vi "SVFA FFT Spectrum Subset (Mag-Phase) (N Ch).vi"(0 "scaled signals [EU]":waveform(dbl)[](array[waveform]), 2 "window":T1=1 items=["None"=0, "Hanning"=1, "Hamming"=2, "Blackman-Harris"=3, "Exact Blackman"=4, "Blackman"=5, "Flat Top"=6, "4 Term B-Harris "=7, "7 Term B-Harris"=8, "Low Sidelobe"=9, "Force"=64, "Exponential"=65, "Blackman Nuttall"=11, "Triangle"=30, "Bartlett-Hanning"=31, "Bohman"=32, "Parzen"=33, "Welch"=34, "Kaiser"=60, "Dolph-Chebyshev"=61, "Gaussian"=62], 3 "frequency range":T3={"start frequency"=1000.0, "stop frequency"=5000.0} {"stop frequency" min=0.0 format="%.2f"; "start frequency" min=0.0 format="%.2f"}, 4 "view":T2={"dB On (T)"=TRUE, "unwrap phase (F)"=FALSE, "convert to degree (T)"=TRUE}, 5 "error in (no error)":errorcluster, 7 "averaging parameters":T10={"averaging mode"=enum."No averaging", "weighting mode"=enum."Exponential", "number of averages"=10, "linear mode"=enum."One shot"} {"number of averages" min=1 step=1}, 9 "restart averaging (F)":bool) -> (11 "averaging done":bool, 13 "averages completed":dbl, 14 "magnitudes [dB EU]":cluster{"f0":dbl, "df":dbl, "magnitude":dbl[]}[](array[cluster]) {"magnitude" format="%.2p"; "df" format="%.2p"; "f0" format="%.2p"}, 15 "magnitude unit labels":string[](array[string]), 16 "phases [degrees]":cluster{"f0":dbl, "df":dbl, "phase":dbl[]}[](array[cluster]) {"phase" format="%.2f"; "df" format="%.2f"; "f0" format="%.2f"}, 17 "phase unit labels":string[](array[string]), 18 "spectrum info":T4[](array[typedef]) {"x-axis units" items=["Time (s)"=0, "Frequency-CB (Hz)"=1, "Frequency-CPB (Hz)"=1248, "Frequency-Arbitrary (Hz)"=2357, "Quefrency (s)"=2, "Revolutions (rev)"=3, "Order"=4, "Speed (RPM)"=11, "Speed (rad/s)"=21, "Index"=65535]; "weighting filter" items=["Linear", "A-weighting", "B-weighting", "C-weighting", "ITU-R 468-4", "Dolby", "CCITT", "C-message", "Wb", "Wc", "Wd", "We", "Wf", "Wh", "Wj", "Wk", "Wm", "AES17 20 kHz lowpass", "AES17 40 kHz lowpass", "AES17 20 kHz highpass", "AES17 40 kHz highpass"]; "dB reference [EU]" format="%.2f"; "engineering units" items=["custom..."=0, "V"=1, "A"=21, "C"=30, "pC"=31, "s"=32, "-"=29, "Pa"=2, "N"=20, "g"=3, "m/s^2"=4, "m/s"=5, "m"=6, "mm/s"=12, "mm"=13, "micron/s"=14, "micron"=15, "in/s^2"=7, "in/s"=8, "in"=9, "mil/s"=10, "mil"=11, "rad/s^2"=16, "rad/s"=17, "rad"=18, "deg/s^2"=26, "deg/s"=27, "deg"=28, "RPM"=22, "cycle/s^2"=23, "Hz"=24, "cycle"=25, "strain"=19]; "spectral info"."window" items=["None "=0, "Hanning"=1, "Hamming"=2, "Blackman-Harris"=3, "Exact Blackman"=4, "Blackman"=5, "Flat Top"=6, "4 Term B-Harris "=7, "7 Term B-Harris"=8, "Low Sidelobe"=9, "Force - Exponential"=10, "Gaussian"=62]}, 19 "error out":errorcluster)   [LabVIEW 2017]
doc: "Computes a subset of the FFT spectrum of <B>scaled signal [EU]</B>. The subset is defined by <B>frequency range</B>. FFT results are returned as magnitude and phase. Each block of data corresponds to a single FFT block and has to be passed individually to this VI. Wire data to the <B>scaled signal [EU]</B> input to determine the polymorphic instance to use or manually select the instance."
uses:
  <vilib>/addons/_NISVFA/_Shared subVIs/Controls/svc_Spectrum Info.ctl
  <vilib>/addons/_NISVFA/_Shared subVIs/Controls/svc_X-Axis Units.ctl
  <vilib>/addons/_NISVFA/_Shared subVIs/Controls/svc_Spectrum Type.ctl
  <vilib>/addons/_NISVFA/_Shared subVIs/Controls/svc_Engineering Units Text Ring.ctl
  <vilib>/addons/_NISVFA/_Shared subVIs/Controls/svc_Weighting Filter Text Ring.ctl
  <vilib>/addons/_NISVFA/_Shared subVIs/Controls/svc_Complimentary Spectrum Units.ctl
  <vilib>/addons/_NISVFA/_Shared subVIs/Controls/svc_Window.ctl
  <vilib>/addons/_NISVFA/_Shared subVIs/Windowing/svfa_Scaled Time Domain Window (1 Ch).vi
  <vilib>/addons/_NISVFA/_Shared subVIs/Spectrum Info/svfa_Build Spectrum Info.vi
  <vilib>/addons/_NISVFA/_Shared subVIs/Spectrum Averaging/svfa_Reset Averaging State Info.vi
  <vilib>/addons/_NISVFA/_Shared subVIs/Spectrum Averaging/svfa_Average Array with Avg Checks (complex) No State.vi
  <vilib>/addons/_NISVFA/_Shared subVIs/Common/svc_Complex to Mag2 Array.vi
  <vilib>/addons/_NISVFA/_Shared subVIs/Spectrum Averaging/svfa_Average Array with Avg Checks (real) No State.vi
  <vilib>/addons/_NISVFA/_Shared subVIs/Windowing/svfa_Scaled Time Domain Window (Array).vi
  <vilib>/addons/_NISVFA/_Shared subVIs/Common/svc_Get SV Channel Info.vi
  <vilib>/addons/_NISVFA/_Shared subVIs/Common/svc_Spectrum Units.vi
  <vilib>/addons/_NISVFA/_Shared subVIs/Spectrum Averaging/svfa_Average Array (complex) No State.vi
  <vilib>/addons/_NISVFA/_Shared subVIs/Spectrum Averaging/svfa_Average Array (real) No State.vi
  <vilib>/Analysis/4window.llb/Force Window.vi
  <vilib>/Analysis/4window.llb/Force Window (DBL).vi
  <vilib>/Analysis/4window.llb/Exponential Window.vi
  <vilib>/Analysis/4window.llb/Exponential Window (DBL).vi
  <vilib>/addons/_NISVFA/_Shared subVIs/Spectrum Averaging/svfa_No Average Array (complex).vi
  <vilib>/addons/_NISVFA/_Shared subVIs/Spectrum Averaging/svfa_Average Array (complex).vi
  <vilib>/addons/_NISVFA/_Shared subVIs/Spectrum Averaging/svfa_No Average Array (real).vi
  <vilib>/addons/_NISVFA/_Shared subVIs/Spectrum Averaging/svfa_Average Array (real).vi
  <vilib>/addons/_NISVFA/_Shared subVIs/Spectrum Averaging/svfa_Peak Hold Array.vi
  <vilib>/addons/_NISVFA/_Shared subVIs/Common/svc_Get Weighting Enum and Labels.vi
  <vilib>/addons/_NISVFA/_Shared subVIs/Common/svc_Unit Label Lexical Class.vi
  <vilib>/addons/_NISVFA/_Shared subVIs/Common/svc_Engineering Units to Unit Label.vi
  <vilib>/addons/_NISVFA/_Shared subVIs/Common/svc_Format Value (DBL).vi
  <vilib>/addons/_NISVFA/_Shared subVIs/Common/svc_Channel Info to Spectrum Info.vi
  <vilib>/addons/_NISVFA/_Shared subVIs/Common/svc_Unit Label to Engineering Units.vi
  <vilib>/Utility/error.llb/Error Cluster From Error Code.vi
  <vilib>/Analysis/0measdsp.llb/Scaled Time Domain Window.vi
  <vilib>/Analysis/0measdsp.llb/Scaled Time Domain Window (DBL).vi
  <vilib>/addons/_NISVFA/_Spectrum Processing/subVIs/svfa_Spectrum Info Window to windowTd Type Def.vi
  <vilib>/addons/_NISVFA/_Shared subVIs/Common/svc_Window Parameters.vi
  <vilib>/addons/_NISVFA/_Shared subVIs/Common/svc_Get Window Info.vi
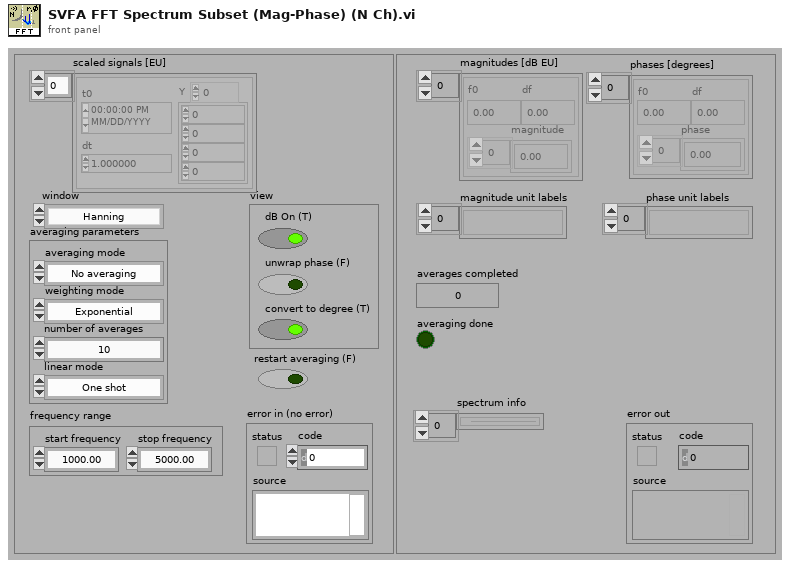
[diagram p1: front panel]
types:
  T1 = typedef "svc_Window.ctl" = u32
  T2 = cluster{"dB On (T)":bool, "unwrap phase (F)":bool, "convert to degree (T)":bool}
  T3 = cluster{"start frequency":dbl, "stop frequency":dbl}
  T4 = typedef "svc_Spectrum Info.ctl" = cluster{"channel name":string, "description":string, "x-axis units":T5, "spectral info":cluster{"spectrum type":T6, "linear/dB":enum16{"linear", "dB"}, "window":u16, "window size":i32, "FFT size":i32}, "engineering units":T7, "custom label":string, "dB reference [EU]":dbl, "peak units":enum16{"rms", "peak", "peak-peak"}, "weighting filter":T8, "spectral density?":bool, "unit label":string, "spectrum skewed?":bool, "complimentary spectrum units":T9}
  T5 = typedef "svc_X-Axis Units.ctl" = u16
  T6 = typedef "svc_Spectrum Type.ctl" = enum16{"FFT Spectrum [complex]", "Amplitude [Magnitude]", "Power [Magnitude^2]", "Cross Spectrum [complex]", "Frequency Response [Complex]"}
  T7 = typedef "svc_Engineering Units Text Ring.ctl" = u16
  T8 = typedef "svc_Weighting Filter Text Ring.ctl" = u16
  T9 = typedef "svc_Complimentary Spectrum Units.ctl" = enum16{"none", "radians", "degrees", "cycles", "imaginary"}
  T10 = cluster{"averaging mode":enum16{"No averaging", "Vector averaging", "RMS averaging", "Peak hold"}, "weighting mode":enum16{"Linear", "Exponential"}, "number of averages":u32, "linear mode":enum16{"One shot", "Auto restart"}}
  T11 = enum16{"Restart processing", "Continue processing", "Skip processing"}
  T12 = cluster{"complex FFT":cdb[], "real FFT":dbl[], "f0":dbl, "df":dbl, "averages completed":dbl, "averaging parameters":cluster{"averaging mode":enum16{"No averaging", "Vector averaging", "RMS averaging", "Peak hold"}, "weighting mode":enum16{"Linear", "Exponential"}, "number of averages":u32, "linear mode":enum16{"One shot", "Auto restart"}}}
  T13 = cluster{"complex FFT":cdb[], "real FFT":dbl[], "f0":dbl, "df":dbl, "averages completed":dbl, "averaging parameters":cluster{"averaging mode":enum16{"No averaging", "Vector averaging", "RMS averaging", "Peak hold"}, "weighting mode":enum16{"Linear", "Exponential"}, "number of averages":u32, "linear mode":enum16{"One shot", "Auto restart"}}}[]
  T14 = enum16{"No averaging", "Vector averaging", "RMS averaging", "Peak hold"}
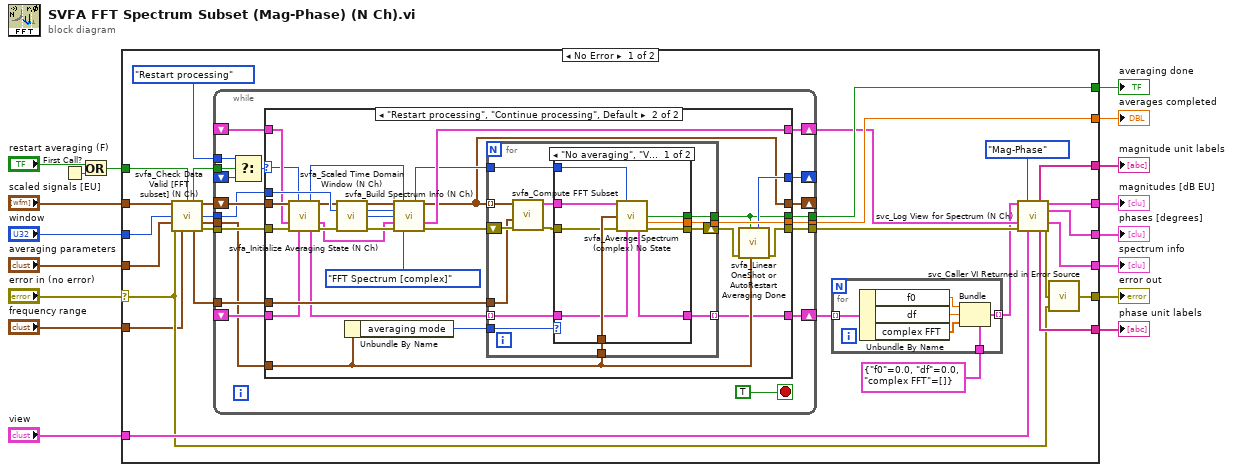
[diagram p0: block diagram]
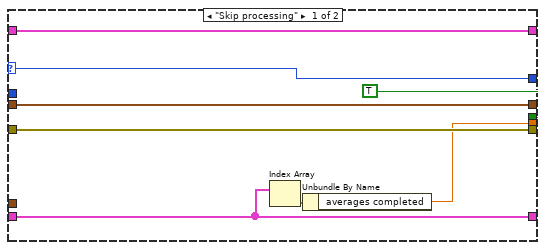
[diagram p2: hidden frame]
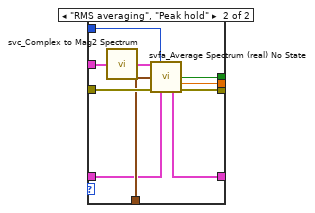
[diagram p3: hidden frame]
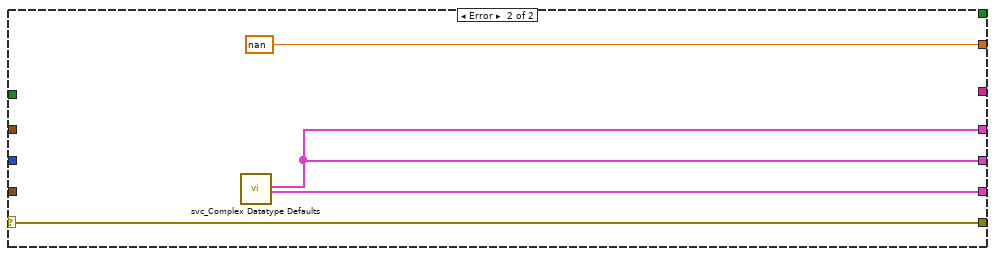
[diagram p4: hidden frame]
diagram:
  n1 = First Call?() -> (First Call?: T/F=w4:bool)
  n2 = Or(x="restart averaging (F)", y=w4) -> (x .or. y?=w2:bool)
  n3 = case shown="No Error" "error in (no error)" {
    selector: "error in (no error)" -> [w35 w144]
    tunnel: w2 -> [w41 _]
    tunnel: [w22 nan ("Averaged So-far")] -> w17
    tunnel: [w36 w144] -> w16
    tunnel: "averaging parameters" -> [w44 _]
    tunnel: "frequency range" -> [w32 _]
    tunnel: "scaled signals [EU]" -> [w46 _]
    tunnel: [w37 w141] -> w5
    tunnel: [w42 _] -> w11
    tunnel: [w45 _] -> w10
    tunnel: [w39 w142] -> w9
    tunnel: [w40 w142] -> w8
    tunnel: [w23 _] -> w7
    tunnel: "view" -> [w43 _]
    tunnel: "window" -> [w34 _]
    frame No Error {
      n4 = call <vilib>:"svfa_Check Data Valid [FFT subset] (N Ch).vi"("scaled signals"=w46, "restart averaging (F)"=w41, "window"=w34, "averaging parameters"=w44, "error in (no error)"=w35, "frequency range in"=w32) -> ("restart averaging"=w25:bool, "dup scaled signals"=w30:waveform(dbl)[], "window"=w29:u16, "dup averaging parameters"=w28:T10, "frequency range out"=w24:T3, "error out"=w27:errorcluster)  [unwired: 4 in]
      n5 = while {
        shift-left: _ -> [w63]
        shift-right: [w64] -> w31
        tunnel: w24 -> [w66]
        tunnel: [w68] -> w22
        tunnel: [w70] -> w23
        tunnel: w27 -> [w71]
        tunnel: [w69] -> w20
        tunnel: w29 -> [w59]
        tunnel: w28 -> [w58]
        shift-right: [w61] -> w21
        shift-left: _ -> [w60]
        shift-right: [w65] -> _
        shift-left: _ -> [w57]
        tunnel: T11."Restart processing" ("t") -> [w56]
        tunnel: w25 -> [w54]
        shift-right: [w53] -> _
        shift-left: w30 -> [w67]
        stop <- TRUE stop-if-true
        n6 = Select(t=w56, s=w54, f=w57) -> (s? t:f=w55:T11)
        n7 = case shown="\"Restart processing\", \"Continue processing\", Default" w55 {
          selector: w55 -> [w77 w82]
          tunnel: w58 -> [_ w106]
          tunnel: [w76 w100] -> w64
          tunnel: w67 -> [w72 w90]
          tunnel: w66 -> [_ w92]
          tunnel: [w77 w105] -> w65
          tunnel: w63 -> [w76 w87]
          tunnel: w59 -> [_ w107]
          tunnel: [w73 w93] -> w61
          tunnel: w60 -> [w73 w89]
          tunnel: [TRUE ("averaging done?") w102] -> w70
          tunnel: [w74 w108] -> w68
          tunnel: [w78 w104] -> w69
          tunnel: w71 -> [w78 w85]
          tunnel: [w72 w80] -> w53
          frame "Skip processing" {
            n8 = Index Array(array=w76) -> (element=w75:T12)  [unwired: 1 in]
            n9 = Unbundle By Name(w75) -> ("averages completed"=w74:dbl)
          }
          frame "Restart processing", "Continue processing", Default {
            n10 = call <vilib>:"svfa_Initialize Averaging State (N Ch).vi"("Windowed Waveform(s)"=w90, "processing control in"=w82, "spectra info in"=w89, "error in (no error)"=w85, "state info"=w87) -> ("processing control out"=w81:T11, "Windowed Waveform(s)"=w88:waveform(dbl)[], "spectra info out"=w83:T4[], "state info"=w86:T13, "error out"=w84:errorcluster)  [unwired: 6 in]
            n11 = call <vilib>:"svfa_Scaled Time Domain Window (N Ch).vi"("Scaled signal(s)"=w88, "window"=w107, "error in (no error)"=w84) -> ("Windowed Waveform(s)"=w97:waveform(dbl)[], "window"=w95:T1, "window length"=w96:i32, "error out"=w98:errorcluster)  [unwired: 8 in, 1 out]
            n12 = Unbundle By Name(w106) -> ("averaging mode"=w101:T14)
            n13 = call <vilib>:"svfa_Build Spectrum Info (N Ch).vi"("scaled signal(s)"=w97, "processing control in"=w81, "window"=w95, "window size"=w96, "spectra info in"=w83, "error in (no error)"=w98, "spectrum type"=svc_Spectrum_Type."FFT Spectrum [complex]" ("spectrum type 2")) -> ("dup processing control"=w91:T11, "dup scaled signals"=w80:waveform(dbl)[], "spectra info out"=w93:T4[], "error out"=w99:errorcluster)  [unwired: 5 in]
            n14 = for {
              tunnel: [w121] -> w108
              tunnel: w106 -> [w120]
              tunnel: [w118] -> w102
              tunnel: w101 -> [w117]
              tunnel: [w116] -> w100 mode=indexing
              tunnel: w92 -> [w114]
              tunnel: w91 -> [w111]
              tunnel: w80 -> [w110] mode=indexing
              tunnel: w86 -> [w109] mode=indexing
              shift-right: [w119] -> w103
              shift-left: w99 -> [w115]
              n15 = call <vilib>:"svfa_Compute FFT Subset.vi"("error in (no error)"=w115, "frequency range"=w114, "windowed signal"=w110) -> ("error out"=w113:errorcluster, "FFT spectrum [Vrms]"=w112:cluster{"f0":dbl, "df":dbl, "spectrum":cdb[]})  [unwired: 7 in]
              n16 = case shown="\"No averaging\", \"Vector averaging\", Default" w117 {
                tunnel: w120 -> [w129 w137]
                tunnel: [w127 w133] -> w119
                tunnel: [w126 w139] -> w118
                tunnel: w112 -> [w130 w134]
                tunnel: w113 -> [w128 w140]
                tunnel: [w124 w138] -> w121
                tunnel: w111 -> [w125 w135]
                tunnel: [w123 w131] -> w116
                tunnel: w109 -> [w122 w132]
                frame "No averaging", "Vector averaging", Default {
                  n17 = call <vilib>:"svfa_Average Spectrum (complex) No State.vi"("spectrum"=w130, "processing control"=w125, "averaging parameters"=w129, "error in (no error)"=w128, "averaging state info in"=w122) -> ("averaging done"=w126:bool, "averages completed"=w124:dbl, "averaging state info out"=w123:T12, "error out"=w127:errorcluster)  [unwired: 5 in, 2 out]
                }
                frame "RMS averaging", "Peak hold" {
                  n18 = call <vilib>:"svc_Complex to Mag2 Spectrum.vi"("complex spectrum"=w134) -> ("power spectrum"=w136:cluster{"f0":dbl, "df":dbl, "spectrum":dbl[]})  [unwired: 4 in]
                  n19 = call <vilib>:"svfa_Average Spectrum (real) No State.vi"("spectrum"=w136, "processing control"=w135, "averaging parameters"=w137, "error in (no error)"=w140, "averaging state info in"=w132) -> ("averaging done"=w139:bool, "averages completed"=w138:dbl, "averaging state info out"=w131:T12, "error out"=w133:errorcluster)  [unwired: 5 in, 2 out]
                }
              }
            }
            n20 = call <vilib>:"svfa_Linear OneShot or AutoRestart Averaging Done.vi"("averaging parameters"=w106, "averaging done"=w102, "error in (no error)"=w103) -> ("error out"=w104:errorcluster, "processing control"=w105:T11)  [unwired: 7 in]
          }
        }
      }
      n21 = for {
        tunnel: w31 -> [w49] mode=indexing
        tunnel: [w48] -> w19 mode=indexing
        tunnel: cluster{"f0":dbl, "df":dbl, "complex FFT":cdb[]} {"f0"=0.0, "df"=0.0, "complex FFT"=[]} ("cluster") -> [w47]
        n22 = Unbundle By Name(w49) -> ("f0"=w52:dbl, "df"=w51:dbl, "complex FFT"=w50:cdb[])
        n23 = Bundle(cluster=w47, "f0"=w52, "df"=w51, "complex FFT"=w50) -> (w48:cluster{"f0":dbl, "df":dbl, "complex FFT":cdb[]})
      }
      n24 = call <vilib>:"svc_Log View for Spectrum (N Ch).vi"("complex spectra"=w19, "View"=enum16{"Mag-Phase", "Real-Imaginary"}."Mag-Phase", "spectra info in"=w21, "error in (no error)"=w20, "view"=w43) -> ("unit label [mag or real]"=w45:string[], "magnitude or real"=w40:cluster{"f0":dbl, "df":dbl, "magnitude":dbl[]}[], "phase or imaginary"=w39:cluster{"f0":dbl, "df":dbl, "magnitude":dbl[]}[], "spectra info out"=w37:T4[], "unit label [phase or imag]"=w42:string[], "error out"=w38:errorcluster)  [unwired: 5 in]
      n25 = call <vilib>:"svc_Caller VI Returned in Error Source.vi"("warning input to caller"=w35, "error in (no error)"=w38) -> ("error out"=w36:errorcluster)  [unwired: 3 in]
    }
    frame Error {
      n26 = call <vilib>:"svc_Complex Datatype Defaults.vi"() -> ("empty array of spectra"=w142:cluster{"f0":dbl, "df":dbl, "magnitude":dbl[]}[], "empty array of spectrum info"=w141:T4[])  [unwired: 11 in, 7 out]
    }
  }
  "averages completed" <- w17
  "error out" <- w16
  "spectrum info" <- w5
  "magnitude unit labels" <- w10
  "phase unit labels" <- w11
  "magnitudes [dB EU]" <- w8
  "phases [degrees]" <- w9
  "averaging done" <- w7
